vi "Get Events.vi"(11 "Create Test Channel View in":refnum<class "Edit Test Channel View.lvclass">) -> (2 "Events":T1, 3 "Create Test Channel View out":refnum<class "Edit Test Channel View.lvclass">)   [LabVIEW 2013, in "Edit Test Channel View.lvlib" / "Edit Test Channel View.lvclass"]
uses:
  Edit Test Channel View.lvclass
  Typedef/Events.ctl
  Edit Test Channel View.lvclass/Edit Test Channel View.ctl
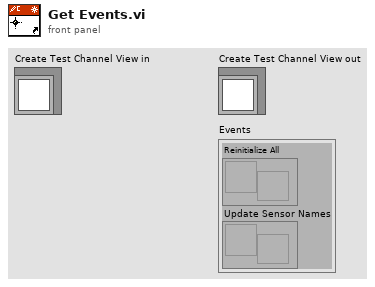
[diagram p1: front panel]
types:
  T1 = typedef "Edit Test Channel View.lvlib/Edit Test Channel View.lvclass/Events.ctl" = cluster{"Reinitialize All":refnum<user-event>, "Update Sensor Names":refnum<user-event>}
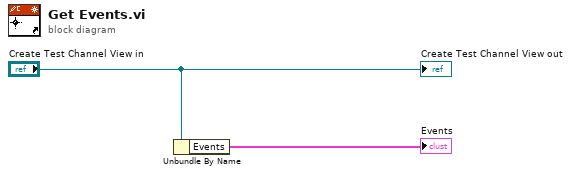
[diagram p0: block diagram]
diagram:
  n1 = Unbundle By Name("Create Test Channel View in") -> ("Events"=→"Events":T1)
  "Create Test Channel View out" <- "Create Test Channel View in"
